vi "Close.vi"(8 "error in (no error)":errorcluster, 11 "UniStableShutter in":refnum<class "UniStableShutter.lvclass">) -> (0 "error out":errorcluster, 3 "UniStableShutter out":refnum<class "UniStableShutter.lvclass">)   [LabVIEW 2016, in "UniStableShutter.lvclass"]
uses:
  UniStableShutter.lvclass
  Shutter.lvclass
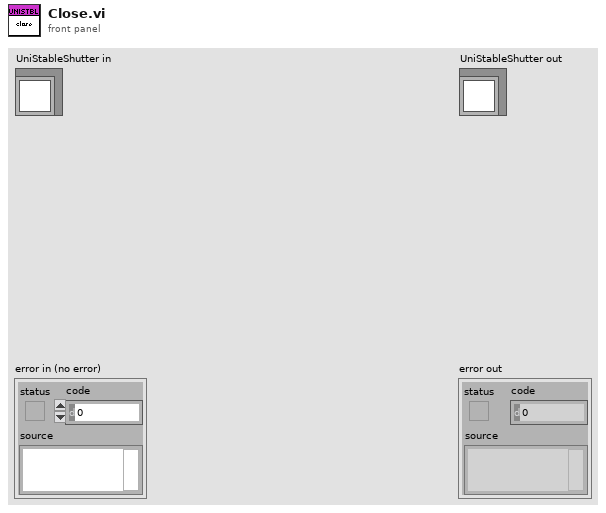
[diagram p1: front panel]
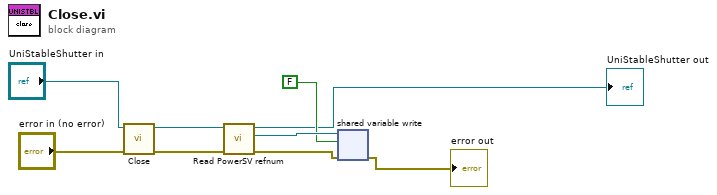
[diagram p0: block diagram]
diagram:
  n1 = call-parent "Close.vi"("error in (no error)"="error in (no error)", "Shutter in"="UniStableShutter in") -> ("error out"=w2:errorcluster, "Shutter out"=w1:refnum<class "UniStableShutter.lvclass">)  [unwired: 8 in]
  n2 = call-dynamic "Read PowerSV refnum.vi"("error in (no error)"=w2, "UniStableShutter in"=w1) -> ("error out"=w5:errorcluster, "PowerSV refnum"=w7:refnum<k21>, "UniStableShutter out"=→"UniStableShutter out":refnum<class "UniStableShutter.lvclass">)  [unwired: 7 in]
  n3 = shared-variable-write(w7, w5, FALSE ("data in")) -> (→"error out":errorcluster)  [unwired: 1 out]
